vi "timer.vi"(8 "error in":errorcluster, 10 "limit":dbl, 11 "timerstatus":T1) -> (0 "error out":errorcluster, 2 "limit out":bool, 3 "elapsed":dbl)   [LabVIEW 2015]
uses:
  timerstatus.ctl
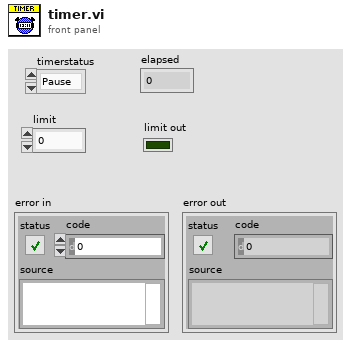
[diagram p1: front panel]
types:
  T1 = typedef "timerstatus.ctl" = enum16{"Pause", "Stop", "Start"}
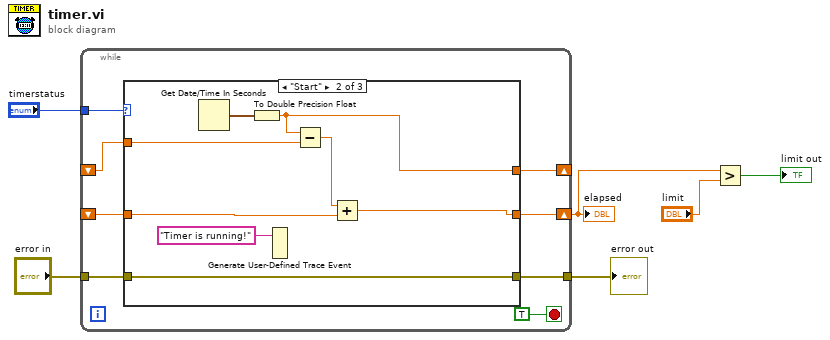
[diagram p0: block diagram]
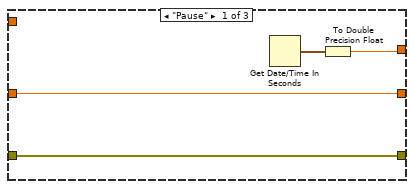
[diagram p2: hidden frame]
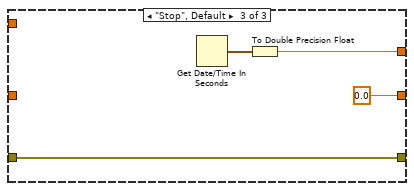
[diagram p3: hidden frame]
diagram:
  n1 = while {
    tunnel: "timerstatus" -> [w13]
    shift-right: [w12] -> _
    shift-left: _ -> [w10]
    shift-right: [w11] -> w1
    shift-left: _ -> [w9]
    tunnel: [w8] -> w3
    tunnel: "error in" -> [w7]
    stop <- TRUE stop-if-true
    n2 = case shown="\"Start\"" w13 {
      tunnel: [w16 w21 w29] -> w12
      tunnel: [w18 w22 0.0] -> w11
      tunnel: w10 -> [_ w25 _]
      tunnel: w9 -> [w18 w23 _]
      tunnel: [w15 w20 w27] -> w8
      tunnel: w7 -> [w15 w20 w27]
      frame "Pause" {
        n3 = Get Date/Time In Seconds() -> (seconds since 1Jan1904=w17:timestamp)
        n4 = To Double Precision Float(number=w17) -> (double precision float=w16:dbl)
      }
      frame "Start" {
        n5 = Get Date/Time In Seconds() -> (seconds since 1Jan1904=w26:timestamp)
        n6 = To Double Precision Float(number=w26) -> (double precision float=w21:dbl)
        n7 = Generate User-Defined Trace Event(2:"Timer is running!" ("trace string")) -> ()  [unwired: 1 in]
        n8 = Subtract(x=w21, y=w25) -> (x-y=w24:dbl)
        n9 = Add(x=w24, y=w23) -> (x+y=w22:dbl)
      }
      frame "Stop", Default {
        n10 = Get Date/Time In Seconds() -> (seconds since 1Jan1904=w30:timestamp)
        n11 = To Double Precision Float(number=w30) -> (double precision float=w29:dbl)
      }
    }
  }
  "elapsed" <- w1
  "error out" <- w3
  n12 = Greater?(x=w1, y="limit") -> (0:→"limit out":bool)
